vi "Find last IFD.vi"(5 "TIFF Data in":u8[](array[numeric])) -> (0 "Location in byte stream of last IFD pointer.  This\nis the word to change if you are adding another page\nto the file.":i32, 1 "IFD locations":u32[](array[numeric]), 2 "Litt/BigEnd":bool)   [LabVIEW 2015, in "Tiff reader.lvlib"]
doc: "This .vi loops through the IFDs in the TIFF data, and finds the IFD locations in the byte stream and also the location in the byte stream of the IFD final pointer (which is needed to append images to the TIFF stack)"
uses:
  Tiff reader.lvlib
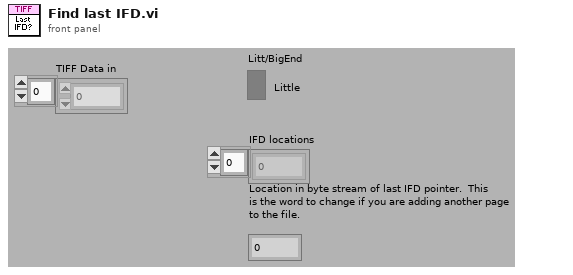
[diagram p1: front panel]
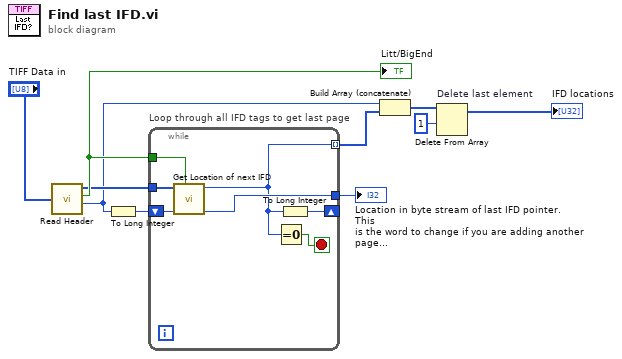
[diagram p0: block diagram]
diagram:
  n1 = call "Read Header.vi"("TIFF Data in"="TIFF Data in") -> ("TIFF Data out"=w7:u8[], "Litt/BigEnd"=w9:bool, "ImFileDirectOffs"=w5:u32)  [unwired: 1 out]
  "Litt/BigEnd" <- w9
  n2 = To Long Integer(number=w5) -> (32bit integer=w1:i32)
  n3 = while "Loop through all IFD tags to get last page" {
    tunnel: w7 -> [w15]
    tunnel: w9 -> [w16]
    shift-right: [w11] -> _
    shift-left: w1 -> [w17]
    tunnel: [w14] -> w10
    tunnel: [w12] -> w6 mode=indexing
    stop <- w13 stop-if-true
    n4 = call "Get Location of next IFD.vi"("Litt/BigEnd"=w16, "Start of current IFD\n(ImFileDirectOffs)"=w17, "Image Data"=w15) -> ("Location in byte stream of Long Word that points to this next IFD"=w14:i32, "Location in byte stream of next IFD if there is a next IFD,\n0 otherwise"=w12:u32)  [unwired: 1 in, 3 out]
    n5 = Equal To 0?(x=w12) -> (x = 0?=w13:bool)
    n6 = To Long Integer(number=w12) -> (32bit integer=w11:i32)
  }
  "Location in byte stream of last IFD pointer.  This\nis the word to change if you are adding another page\nto the file." <- w10
  n7 = Build Array (concatenate)(w5, w6) -> (w4:u32[])
  n8 = Delete From Array "Delete last element"(array=w4, length=1) -> (array with subset deleted=→"IFD locations":u32[])  [unwired: 1 in, 1 out]
